vi "Validate_Simulation.vi"() -> ()   [LabVIEW 2020, in "AbstractDMM.lvlib" / "Keysight_34401A-DMM.lvclass"]
uses:
  Keysight_34401A-DMM.lvclass
  <instrlib>/Agilent 34401/Public/Data/Read (Single Point).vi
  Session Factory/Session Factory.lvclass
  <vilib>/MeasurementLink/MeasurementLink Instrument/ISession Factory/Remote Connection Options.ctl
  <vilib>/MeasurementLink/MeasurementLink Instrument/ISession Factory/ISession Factory.lvclass
  <vilib>/MeasurementLink/MeasurementLink Instrument/ISession Factory/Session Initialization Parameters.ctl
  <instrlib>/Agilent 34401/Agilent 34401.lvlib
  <vilib>/MeasurementLink/MeasurementLink Instrument/ISession Factory/Initialize and Close Session Behavior.ctl
panel:
  out "error out":errorcluster
  out "Measurement":dbl
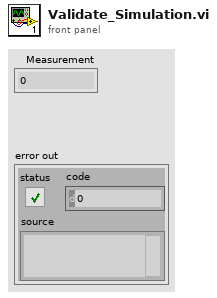
[diagram p1: front panel]
types:
  T1 = typedef "MeasurementLink Instrument.lvlib/ISession Factory.lvclass/Initialize and Close Session Behavior.ctl" = enum16{"Initialize and Close", "Attach and Detach", "Initialize and Detach", "Attach and Close"}
  T2 = typedef "MeasurementLink Instrument.lvlib/ISession Factory.lvclass/Session Initialization Parameters.ctl" = cluster{"resource name":string, "session name":string}
  T3 = typedef "MeasurementLink Instrument.lvlib/ISession Factory.lvclass/Remote Connection Options.ctl" = cluster{"session name":string, "address":string, "port":u32}
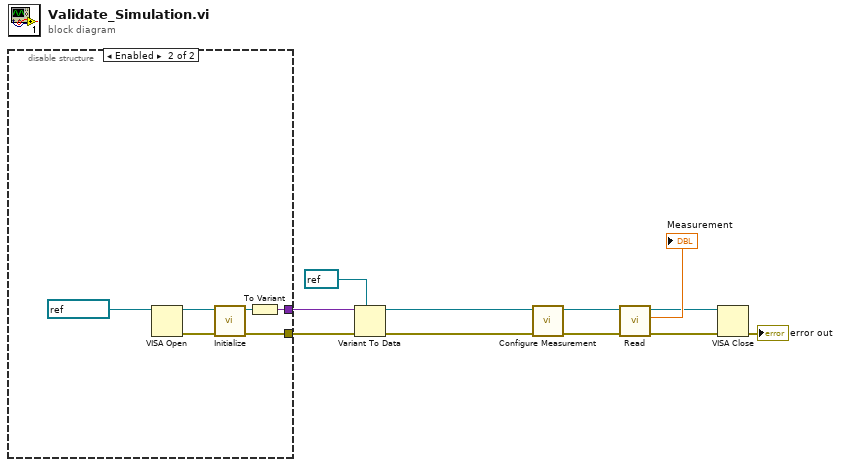
[diagram p0: block diagram]
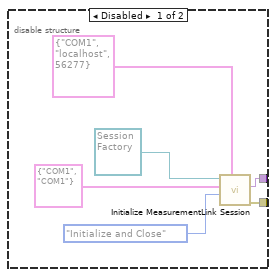
[diagram p2: hidden frame]
diagram:
  n1 = disable-structure shown="Enabled" {
    disable-tunnel: [w14 w21] -> w9
    disable-tunnel: [w13 w18] -> w7
    frame Disabled {
      n2 = call-dynamic "Initialize MeasurementLink Session.vi"("remote connection options"=T3 {"session name"="COM1", "address"="localhost", "port"=56277}, "initialize session behavior"=Initialize_and_Close_Session_Behavior."Initialize and Close", "session initialization parameters"=T2 {"resource name"="COM1", "session name"="COM1"}, "session factory in"=refnum<class "Session Factory.lvclass"> refnum) -> ("error out"=w14:errorcluster, "session out"=w13:variant)  [unwired: 5 in, 1 out]
    }
    frame Enabled {
      n3 = VISA Open(VISA resource name=refnum<visa-resource-name> "COM1") -> (VISA resource name=w20:refnum<visa-resource-name>, error out=w22:errorcluster)  [unwired: 4 in]
      n4 = call <instrlib>:"Initialize.vi"("error in (no error)"=w22, "VISA resource name"=w20) -> ("error out"=w21:errorcluster, "VISA resource name out"=w19:refnum<visa-resource-name>)  [unwired: 8 in]
      n5 = To Variant(anything=w19) -> (Variant=w18:variant)
    }
  }
  n6 = Variant To Data(error in=w9, type=refnum<visa-resource-name> refnum ("VISA resource name"), Variant=w7) -> (data=w2:refnum<visa-resource-name>, error out=w8:errorcluster)
  n7 = call <instrlib>:"Configure Measurement.vi"("error in (no error)"=w8, "VISA resource name"=w2) -> ("error out"=w10:errorcluster, "VISA resource name out"=w11:refnum<visa-resource-name>)  [unwired: 8 in]
  n8 = call-poly <instrlib>:"Read.vi"("error in (no error)"=w10, "VISA resource name"=w11) -> ("error out"=w3:errorcluster, "Measurement"=→"Measurement":dbl, "VISA resource name out"=w4:refnum<visa-resource-name>)  [unwired: 7 in]
  n9 = VISA Close(VISA resource name=w4, error in (no error)=w3) -> (error out=→"error out":errorcluster)
